vi "QCA9984 Write Memory.vi"(4 "Commit?":bool, 5 "Operation":T2(ring), 6 "Write?":bool, 8 "error in":errorcluster, 10 "Memory":T1={"WIFI"={"Mac Address in"="\u0001\u0000\u0000Àÿî", "regDmn in"=106, "WIFI VID"=5772, "WIFI DID"=62, "SVID"=6058, "SSID"=12356}, "BT"={"BD Address in"="\u0019Ï^ç ¦", "BT PID VID Address"=17, "PID VID Value"=0}} {"BT"."PID VID Value" format="%x"; "BT"."BT PID VID Address" format="%x"; "WIFI"."SSID" format="%x"; "WIFI"."SVID" format="%x"; "WIFI"."WIFI DID" format="%x"; "WIFI"."WIFI VID" format="%x"; "WIFI"."regDmn in" format="%x"}, 11 "_hResourceContext in":u32) -> (0 "error out":errorcluster, 2 "Mac Address out":string, 3 "_hResourceContext out":u32)   [LabVIEW 2013]
uses:
  QCAWLAN_DLL.lvlib
panel:
  out "OTP Value out":u32[](array[numeric]) format="%x"
  in  "OTP Value":u32[](array[numeric]) format="%x"
  in  "OTP Address":u32[](array[numeric])
  out "BT PID VID Value out":u32 format="%x"
  out "SVID out":u32 format="%x"
  out "SSID out":u32 format="%x"
  out "WIFI DID out":u32 format="%x"
  out "WIFI VID out":u32 format="%x"
  out "BD Address out":string
  out "regDmn out":u32 format="%x"
  # "Write"
  # "Read"
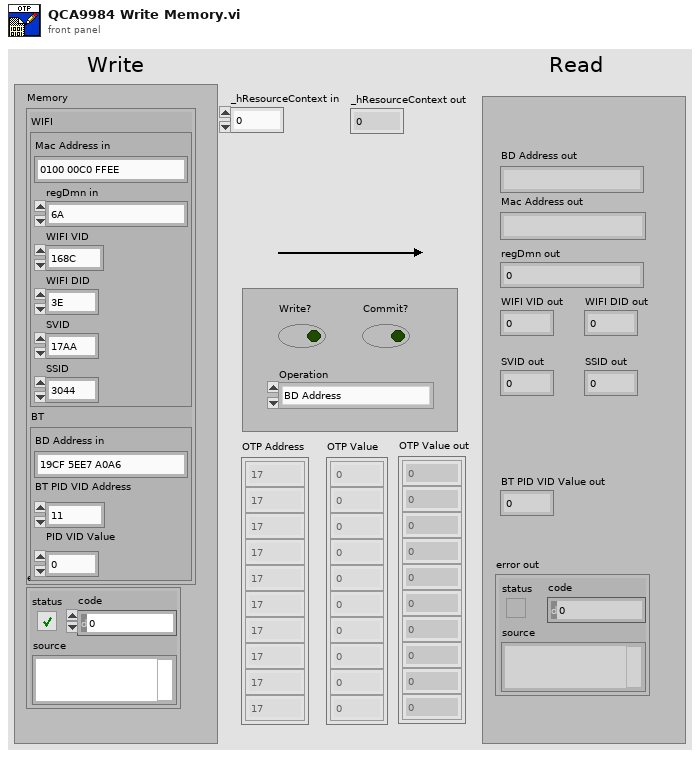
[diagram p1: front panel]
types:
  T1 = cluster{"WIFI":cluster{"Mac Address in":string, "regDmn in":u32, "WIFI VID":u32, "WIFI DID":u32, "SVID":u32, "SSID":u32}, "BT":cluster{"BD Address in":string, "BT PID VID Address":u32, "PID VID Value":u32}}
  T2 = enum16{"BD Address", "Mac Address", "Reg Domain", "WIFI VID", "WIFI DID", "SSID", "SVID", "OTP", "BT PID VID", "Dump OTP to File", "None"}
  T3 = cluster{"iTemplateNum":u8, "iWriteOption":u8, "iMemSize":u32, "iCompress":u8, "iOverwrite":u8, "iSectionMask":i32[]}
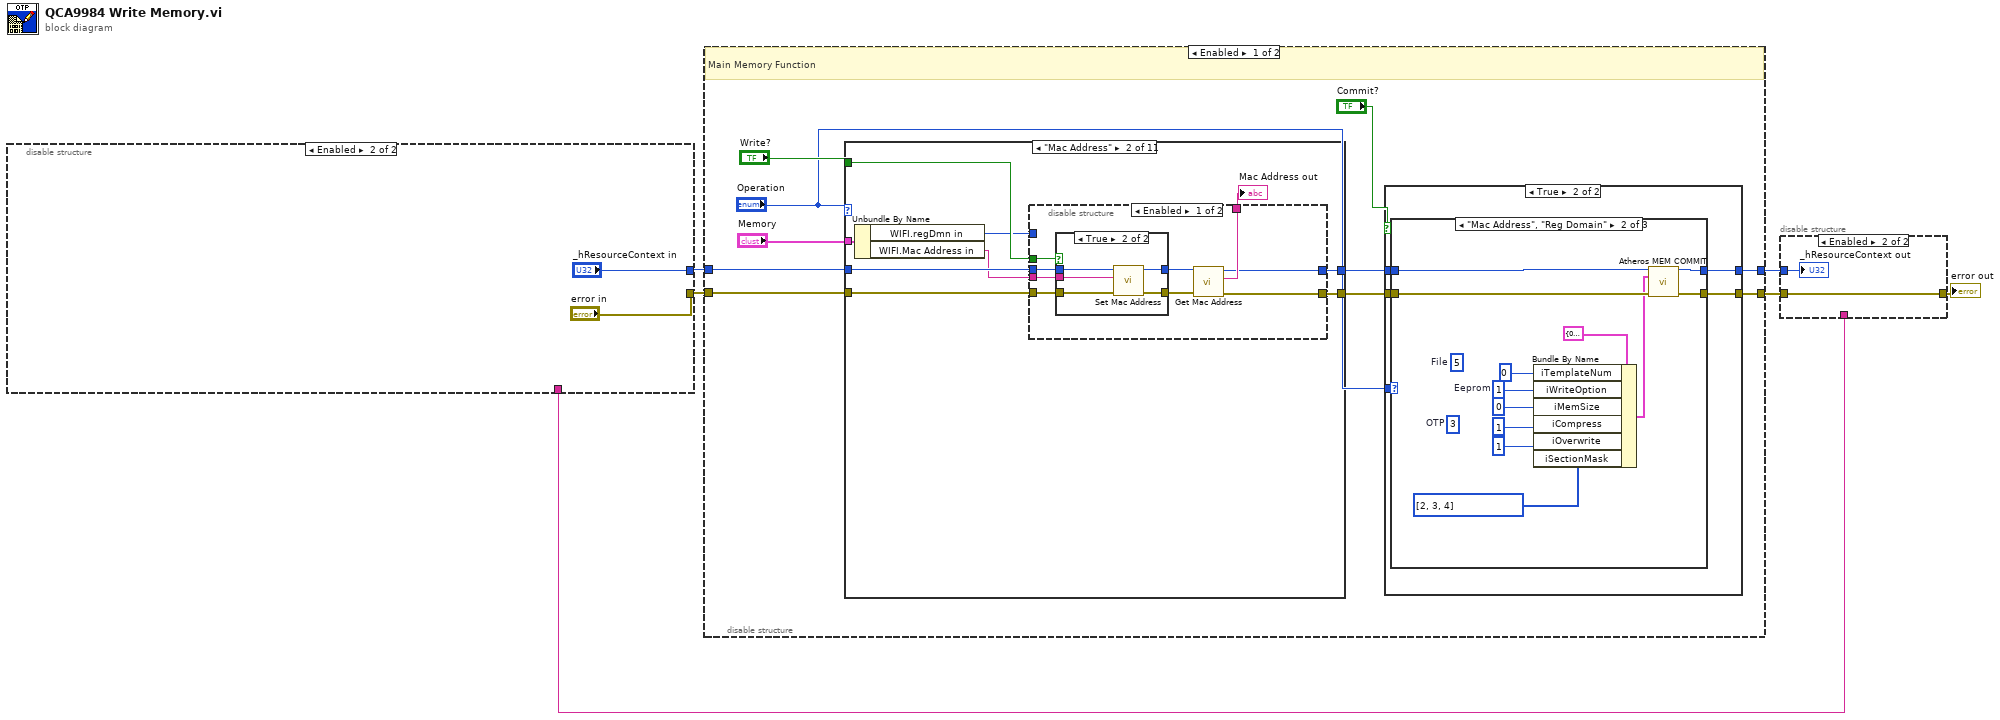
[diagram p0: block diagram]
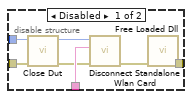
[diagram p2: hidden frame]
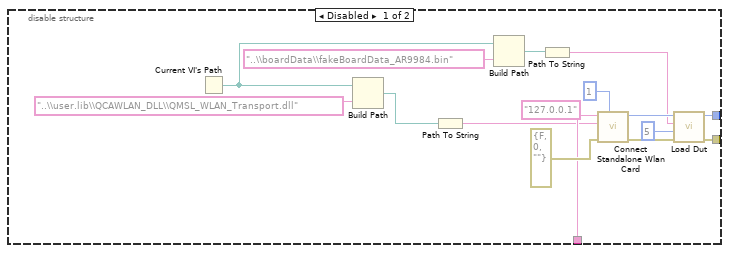
[diagram p3: hidden frame]
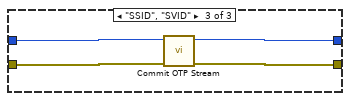
[diagram p6: hidden frame]
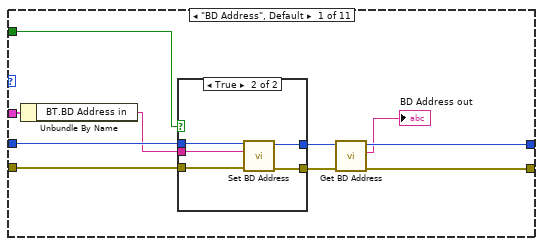
[diagram p7: hidden frame]
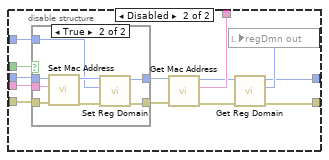
[diagram p10: hidden frame]
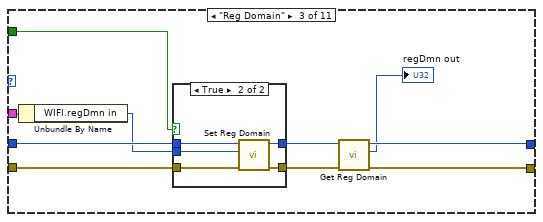
[diagram p12: hidden frame]
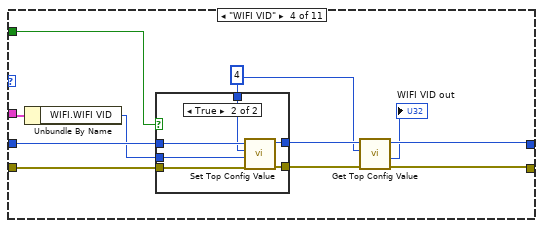
[diagram p14: hidden frame]
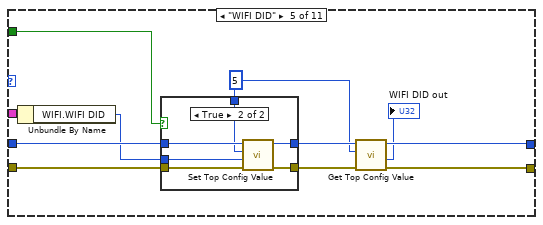
[diagram p16: hidden frame]
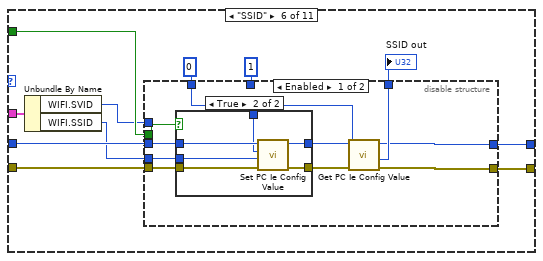
[diagram p18: hidden frame]
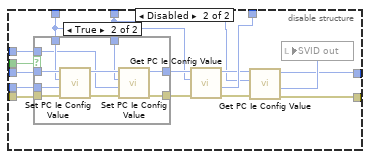
[diagram p20: hidden frame]
diagram:
  n1 = disable-structure shown="Enabled" {
    disable-tunnel: [w19 _] -> w5
    disable-tunnel: [w18 "error in"] -> w4
    disable-tunnel: [w17 "_hResourceContext in"] -> w3
    frame Disabled {
      w19 = "127.0.0.1" ("USER_DUT_IP")
      n2 = Current VI's Path() -> (path=w12:path)
      n3 = Build Path(base path=w12, name or relative path="..\\user.lib\\QCAWLAN_DLL\\QMSL_WLAN_Transport.dll") -> (appended path=w14:path)
      n4 = Path To String(path=w14) -> (string=w8:string)
      n5 = Build Path(base path=w12, name or relative path="..\\boardData\\fakeBoardData_AR9984.bin") -> (appended path=w10:path)
      n6 = Path To String(path=w10) -> (string=w7:string)
      n7 = call "Connect Standalone Wlan Card.vi"("DutNum"=1, "error in (no error)"=errorcluster {"status"=FALSE, "code"=0, "source"=""}, "dllPath"=w8, "USER_DUT_IP"=w19) -> ("error out"=w21:errorcluster, "function return"=w16:u32)  [unwired: 2 in, 4 out]
      n8 = call "Load Dut.vi"("error in (no error)"=w21, "iNVMemOption"=5, "USER_BIN_FILE"=w7, "_hResourceContext"=w16) -> ("error out"=w18:errorcluster, "_hResourceContext out"=w17:u32)  [unwired: 4 in, 2 out]
    }
    frame Enabled {
    }
  }
  n9 = disable-structure shown="Enabled" {
    disable-tunnel: w4 -> [w33 w321]
    disable-tunnel: w3 -> [w32 w322]
    disable-tunnel: [w26 w321] -> w2
    disable-tunnel: [w25 w322] -> w1
    frame Enabled {
      # "Main Memory Function"
      n10 = case shown="\"Mac Address\"" "Operation" {
        tunnel: w33 -> [w68 w84 w133 w151 w170 w189 w245 w264 w290 w318 w319]
        tunnel: [w65 w79 w130 w148 w167 w183 w237 w266 w288 w317 w319] -> w31
        tunnel: w32 -> [w67 w83 w132 w150 w169 w188 w244 w263 w289 w315 w320]
        tunnel: [w63 w80 w128 w146 w165 w184 w236 w265 w287 w316 w320] -> w30
        tunnel: "Write?" -> [w61 w81 w126 w143 w162 w185 w239 w262 w286 _ _]
        tunnel: "Memory" -> [w60 w78 w125 w142 w161 w182 _ _ w285 _ _]
        frame "BD Address", Default {
          n11 = Unbundle By Name(w60) -> ("BT.BD Address in"=w59:string)
          n12 = case shown="True" w61 {
            tunnel: w68 -> [w70 w75]
            tunnel: w67 -> [w69 w74]
            tunnel: [w70 w73] -> w66
            tunnel: [w69 w72] -> w64
            tunnel: w59 -> [_ w71]
            frame False {
            }
            frame True {
              n13 = call "Set BD Address.vi"("error in (no error)"=w75, "addr"=w71, "_hResourceContext"=w74) -> ("error out"=w73:errorcluster, "_hResourceContext out"=w72:u32)  [unwired: 6 in, 1 out]
            }
          }
          n14 = call "Get BD Address.vi"("error in (no error)"=w66, "_hResourceContext"=w64) -> ("error out"=w65:errorcluster, "addr out"=→"BD Address out":string, "_hResourceContext out"=w63:u32)  [unwired: 7 in]
        }
        frame "Mac Address" {
          n15 = Unbundle By Name(w78) -> ("WIFI.regDmn in"=w76:u32, "WIFI.Mac Address in"=w77:string)
          n16 = disable-structure shown="Enabled" {
            disable-tunnel: w84 -> [w93 w108]
            disable-tunnel: w83 -> [w92 w110]
            disable-tunnel: [w89 w106] -> w82
            disable-tunnel: w81 -> [w88 w111]
            disable-tunnel: [w87 w102] -> w80
            disable-tunnel: [w86 w101] -> w79
            disable-tunnel: w77 -> [w85 w109]
            disable-tunnel: w76 -> [_ w107]
            frame Enabled {
              n17 = case shown="True" w88 {
                tunnel: w93 -> [w94 w100]
                tunnel: w92 -> [w95 w99]
                tunnel: [w94 w98] -> w91
                tunnel: [w95 w97] -> w90
                tunnel: w85 -> [_ w96]
                frame False {
                }
                frame True {
                  n18 = call "Set Mac Address.vi"("error in (no error)"=w100, "addr"=w96, "_hResourceContext"=w99) -> ("error out"=w98:errorcluster, "_hResourceContext out"=w97:u32)  [unwired: 6 in, 1 out]
                }
              }
              n19 = call "Get Mac Address.vi"("error in (no error)"=w91, "_hResourceContext"=w90) -> ("error out"=w86:errorcluster, "buffer out"=w89:string, "_hResourceContext out"=w87:u32)  [unwired: 7 in]
            }
            frame Disabled {
              n20 = case shown="True" w111 {
                tunnel: w108 -> [w114 w123]
                tunnel: w110 -> [w115 w122]
                tunnel: [w114 w119] -> w113
                tunnel: [w115 w117] -> w112
                tunnel: w109 -> [_ w121]
                tunnel: w107 -> [_ w116]
                frame False {
                }
                frame True {
                  n21 = call "Set Mac Address.vi"("error in (no error)"=w123, "addr"=w121, "_hResourceContext"=w122) -> ("error out"=w120:errorcluster, "_hResourceContext out"=w118:u32)  [unwired: 6 in, 1 out]
                  n22 = call "Set Reg Domain.vi"("error in (no error)"=w120, "regDmn"=w116, "_hResourceContext"=w118) -> ("error out"=w119:errorcluster, "_hResourceContext out"=w117:u32)  [unwired: 6 in, 1 out]
                }
              }
              n23 = call "Get Mac Address.vi"("error in (no error)"=w113, "_hResourceContext"=w112) -> ("error out"=w105:errorcluster, "buffer out"=w106:string, "_hResourceContext out"=w104:u32)  [unwired: 7 in]
              n24 = call "Get Reg Domain.vi"("error in (no error)"=w105, "_hResourceContext"=w104) -> ("error out"=w101:errorcluster, "regDmn out"=w103:u32, "_hResourceContext out"=w102:u32)  [unwired: 7 in]
              n25 = local write "regDmn out"(w103) -> ()
            }
          }
          "Mac Address out" <- w82
        }
        frame "Reg Domain" {
          n26 = Unbundle By Name(w125) -> ("WIFI.regDmn in"=w124:u32)
          n27 = case shown="True" w126 {
            tunnel: w133 -> [w134 w140]
            tunnel: w132 -> [w135 w139]
            tunnel: [w134 w138] -> w131
            tunnel: [w135 w137] -> w129
            tunnel: w124 -> [_ w136]
            frame False {
            }
            frame True {
              n28 = call "Set Reg Domain.vi"("error in (no error)"=w140, "regDmn"=w136, "_hResourceContext"=w139) -> ("error out"=w138:errorcluster, "_hResourceContext out"=w137:u32)  [unwired: 6 in, 1 out]
            }
          }
          n29 = call "Get Reg Domain.vi"("error in (no error)"=w131, "_hResourceContext"=w129) -> ("error out"=w130:errorcluster, "regDmn out"=→"regDmn out":u32, "_hResourceContext out"=w128:u32)  [unwired: 7 in]
        }
        frame "WIFI VID" {
          w145 = u32 4 ("action")
          n30 = Unbundle By Name(w142) -> ("WIFI.WIFI VID"=w141:u32)
          n31 = case shown="True" w143 {
            tunnel: w151 -> [w152 w159]
            tunnel: w150 -> [w153 w158]
            tunnel: [w152 w157] -> w149
            tunnel: [w153 w156] -> w147
            tunnel: w145 -> [_ w155]
            tunnel: w141 -> [_ w154]
            frame False {
            }
            frame True {
              n32 = call "Set Top Config Value.vi"("error in (no error)"=w159, "value"=w154, "action"=w155, "_hResourceContext"=w158) -> ("error out"=w157:errorcluster, "_hResourceContext out"=w156:u32)  [unwired: 6 in]
            }
          }
          n33 = call "Get Top Config Value.vi"("error in (no error)"=w149, "action"=w145, "_hResourceContext"=w147) -> ("error out"=w148:errorcluster, "value out"=→"WIFI VID out":u32, "_hResourceContext out"=w146:u32)  [unwired: 6 in]
        }
        frame "WIFI DID" {
          w164 = u32 5 ("action")
          n34 = Unbundle By Name(w161) -> ("WIFI.WIFI DID"=w160:u32)
          n35 = case shown="True" w162 {
            tunnel: w170 -> [w171 w178]
            tunnel: w169 -> [w172 w177]
            tunnel: [w171 w176] -> w168
            tunnel: [w172 w175] -> w166
            tunnel: w164 -> [_ w174]
            tunnel: w160 -> [_ w173]
            frame False {
            }
            frame True {
              n36 = call "Set Top Config Value.vi"("error in (no error)"=w178, "value"=w173, "action"=w174, "_hResourceContext"=w177) -> ("error out"=w176:errorcluster, "_hResourceContext out"=w175:u32)  [unwired: 6 in]
            }
          }
          n37 = call "Get Top Config Value.vi"("error in (no error)"=w168, "action"=w164, "_hResourceContext"=w166) -> ("error out"=w167:errorcluster, "value out"=→"WIFI DID out":u32, "_hResourceContext out"=w165:u32)  [unwired: 6 in]
        }
        frame "SSID" {
          n38 = Unbundle By Name(w182) -> ("WIFI.SVID"=w180:u32, "WIFI.SSID"=w181:u32)
          n39 = disable-structure shown="Enabled" {
            disable-tunnel: w189 -> [w199 w220]
            disable-tunnel: w188 -> [w198 w219]
            disable-tunnel: u32 0 ("action") -> [w191 w215]
            disable-tunnel: [w195 w214] -> w186
            disable-tunnel: w185 -> [w194 w218]
            disable-tunnel: [w193 w209] -> w184
            disable-tunnel: [w192 w208] -> w183
            disable-tunnel: w181 -> [w190 w217]
            disable-tunnel: w180 -> [_ w216]
            disable-tunnel: u32 1 ("action") -> [_ w211]
            frame Enabled {
              n40 = case shown="True" w194 {
                tunnel: w199 -> [w200 w207]
                tunnel: w198 -> [w201 w206]
                tunnel: [w200 w205] -> w197
                tunnel: [w201 w204] -> w196
                tunnel: w191 -> [_ w203]
                tunnel: w190 -> [_ w202]
                frame False {
                }
                frame True {
                  n41 = call "Set PC Ie Config Value.vi"("error in (no error)"=w207, "value"=w202, "action"=w203, "_hResourceContext"=w206) -> ("error out"=w205:errorcluster, "_hResourceContext out"=w204:u32)  [unwired: 6 in]
                }
              }
              n42 = call "Get PC Ie Config Value.vi"("error in (no error)"=w197, "action"=w191, "_hResourceContext"=w196) -> ("error out"=w192:errorcluster, "value out"=w195:u32, "_hResourceContext out"=w193:u32)  [unwired: 6 in]
            }
            frame Disabled {
              n43 = case shown="True" w218 {
                tunnel: w220 -> [w223 w234]
                tunnel: w219 -> [w224 w233]
                tunnel: [w223 w228] -> w222
                tunnel: [w224 w227] -> w221
                tunnel: w215 -> [_ w232]
                tunnel: w217 -> [_ w231]
                tunnel: w216 -> [_ w226]
                tunnel: w211 -> [_ w225]
                frame False {
                }
                frame True {
                  n44 = call "Set PC Ie Config Value.vi"("error in (no error)"=w234, "value"=w231, "action"=w232, "_hResourceContext"=w233) -> ("error out"=w230:errorcluster, "_hResourceContext out"=w229:u32)  [unwired: 6 in]
                  n45 = call "Set PC Ie Config Value.vi"("error in (no error)"=w230, "value"=w226, "action"=w225, "_hResourceContext"=w229) -> ("error out"=w228:errorcluster, "_hResourceContext out"=w227:u32)  [unwired: 6 in]
                }
              }
              n46 = call "Get PC Ie Config Value.vi"("error in (no error)"=w222, "action"=w215, "_hResourceContext"=w221) -> ("error out"=w213:errorcluster, "value out"=w214:u32, "_hResourceContext out"=w212:u32)  [unwired: 6 in]
              n47 = call "Get PC Ie Config Value.vi"("error in (no error)"=w213, "action"=w211, "_hResourceContext"=w212) -> ("error out"=w208:errorcluster, "value out"=w210:u32, "_hResourceContext out"=w209:u32)  [unwired: 6 in]
              n48 = local write "SVID out"(w210) -> ()
            }
          }
          "SSID out" <- w186
        }
        frame "SVID" {
          w241 = u32 1 ("action")
          n49 = case shown="True" w239 {
            tunnel: w245 -> [w252 w258]
            tunnel: w244 -> [w253 w257]
            tunnel: [w252 w256] -> w243
            tunnel: [w253 w255] -> w242
            tunnel: w241 -> [_ w254]
            frame False {
            }
            frame True {
              n50 = call "Set PC Ie Config Value.vi"("error in (no error)"=w258, "action"=w254, "_hResourceContext"=w257) -> ("error out"=w256:errorcluster, "_hResourceContext out"=w255:u32)  [unwired: 7 in]
            }
          }
          n51 = call "Get PC Ie Config Value.vi"("error in (no error)"=w243, "action"=w241, "_hResourceContext"=w242) -> ("error out"=w238:errorcluster, "value out"=→"SVID out":u32, "_hResourceContext out"=w235:u32)  [unwired: 6 in]
          n52 = disable-structure shown="Enabled" {
            disable-tunnel: w238 -> [w249 w250]
            disable-tunnel: [w248 w250] -> w237
            disable-tunnel: [w247 w251] -> w236
            disable-tunnel: w235 -> [w246 w251]
            frame Disabled {
              n53 = call "Commit OTP Stream.vi"("error in (no error)"=w249, "_hResourceContext"=w246) -> ("error out"=w248:errorcluster, "_hResourceContext out"=w247:u32)  [unwired: 8 in]
            }
            frame Enabled {
            }
          }
        }
        frame "OTP" {
          n54 = for {
            tunnel: [w276] -> w266
            tunnel: [w275] -> w265
            tunnel: w264 -> [w274]
            tunnel: w263 -> [w272]
            tunnel: w262 -> [w270]
            tunnel: [w269] -> w259 mode=indexing
            tunnel: "OTP Value" -> [w268] mode=indexing
            tunnel: "OTP Address" -> [w267] mode=indexing
            n55 = case shown="True" w270 {
              tunnel: w274 -> [w277 w284]
              tunnel: [w277 w283] -> w273
              tunnel: w272 -> [w278 w282]
              tunnel: [w278 w281] -> w271
              tunnel: w267 -> [_ w279]
              tunnel: w268 -> [_ w280]
              frame False {
              }
              frame True {
                n56 = call "Write OTP Location.vi"("error in (no error)"=w284, "value"=w280, "address"=w279, "_hResourceContext"=w282) -> ("error out"=w283:errorcluster, "_hResourceContext out"=w281:u32)  [unwired: 6 in]
              }
            }
            n57 = call "Read OTP Location.vi"("error in (no error)"=w273, "address"=w267, "_hResourceContext"=w271) -> ("error out"=w276:errorcluster, "value out"=w269:u32, "_hResourceContext out"=w275:u32)  [unwired: 6 in]
          }
          "OTP Value out" <- w259
        }
        frame "BT PID VID" {
          n58 = disable-structure shown="Disabled" {
            disable-tunnel: w290 -> [w297 w313]
            disable-tunnel: w289 -> [w296 w312]
            disable-tunnel: [w295 w313] -> w288
            disable-tunnel: [w294 w312] -> w287
            disable-tunnel: w286 -> [w293 _]
            disable-tunnel: w285 -> [w291 _]
            frame Disabled {
              n59 = Unbundle By Name(w291) -> ()  [unwired: 2 out]
              n60 = for {
                tunnel: w297 -> [w305]
                tunnel: w296 -> [w304]
                tunnel: [w302] -> w295
                tunnel: [w301] -> w294
                tunnel: w293 -> [w299]
                tunnel: [w298] -> w292 mode=indexing
                n61 = case shown="True" w299 {
                  tunnel: w305 -> [w306 w311]
                  tunnel: w304 -> [w307 w310]
                  tunnel: [w306 w309] -> w303
                  tunnel: [w307 w308] -> w300
                  frame False {
                  }
                  frame True {
                    n62 = call "Write OTP Location.vi"("error in (no error)"=w311, "_hResourceContext"=w310) -> ("error out"=w309:errorcluster, "_hResourceContext out"=w308:u32)  [unwired: 8 in]
                  }
                }
                n63 = call "Read OTP Location.vi"("error in (no error)"=w303, "_hResourceContext"=w300) -> ("error out"=w302:errorcluster, "value out"=w298:u32, "_hResourceContext out"=w301:u32)  [unwired: 7 in]
              }
              "BT PID VID Value out" <- w292
            }
            frame Enabled {
            }
          }
        }
        frame "Dump OTP to File" {
          n64 = call "Dump OTP To File.vi"("error in (no error)"=w318, "filename"="C:\\Log\\otpRawContents.txt", "_hResourceContext"=w315) -> ("error out"=w317:errorcluster, "_hResourceContext out"=w316:u32)  [unwired: 6 in, 1 out]
        }
        frame "None" {
        }
      }
      n65 = case shown="True" "Commit?" {
        tunnel: [w34 w36] -> w26
        tunnel: [w35 w37] -> w25
        tunnel: w31 -> [w34 w40]
        tunnel: w30 -> [w35 w39]
        tunnel: "Operation" -> [_ w38]
        frame False {
        }
        frame True {
          n66 = case shown="\"Mac Address\", \"Reg Domain\"" w38 {
            tunnel: w40 -> [w41 w54 w57]
            tunnel: [w41 w53 w55] -> w36
            tunnel: w39 -> [w42 w52 w58]
            tunnel: [w42 w51 w56] -> w37
            frame Default {
            }
            frame "Mac Address", "Reg Domain" {
              (unwired) u8 5  # File
              (unwired) u8 3  # OTP
              w46 = u8 1  # Eeprom
              n67 = Bundle By Name(cluster=T3 {"iTemplateNum"=0, "iWriteOption"=0, "iMemSize"=0, "iCompress"=0, "iOverwrite"=0, "iSectionMask"=[]} ("CommitMemPara"), "iTemplateNum"=u8 0, "iWriteOption"=w46, "iMemSize"=u32 0, "iCompress"=u8 1, "iOverwrite"=u8 1, "iSectionMask"=i32[] [2, 3, 4]) -> (w43:T3)
              n68 = call "Atheros MEM COMMIT.vi"("_hResourceContext"=w52, "CommitMemPara"=w43, "error in (no error)"=w54) -> ("_hResourceContext out"=w51:u32, "error out"=w53:errorcluster)  [unwired: 10 in, 1 out]
            }
            frame "SSID", "SVID" {
              n69 = call "Commit OTP Stream.vi"("error in (no error)"=w57, "_hResourceContext"=w58) -> ("error out"=w55:errorcluster, "_hResourceContext out"=w56:u32)  [unwired: 8 in]
            }
          }
        }
      }
    }
    frame Disabled {
    }
  }
  n70 = disable-structure shown="Enabled" {
    disable-tunnel: [w328 w331] -> w6
    disable-tunnel: w5 -> [w327 _]
    disable-tunnel: w2 -> [w326 w331]
    disable-tunnel: w1 -> [w323 w330]
    frame Disabled {
      n71 = call "Close Dut.vi"("error in (no error)"=w326, "_hResourceContext"=w323) -> ("error out"=w325:errorcluster, "_hResourceContext out"=w324:u32)  [unwired: 7 in, 1 out]
      n72 = call "Disconnect Standalone Wlan Card.vi"("error in (no error)"=w325, "USER_DUT_IP"=w327, "_hResourceContext"=w324) -> ("error out"=w329:errorcluster)  [unwired: 5 in, 3 out]
      n73 = call "Free Loaded Dll.vi"("error in (no error)"=w329) -> ("error out"=w328:errorcluster)  [unwired: 9 in, 1 out]
    }
    frame Enabled {
      "_hResourceContext out" <- w330
    }
  }
  "error out" <- w6
